vi "输入数据解析.vi"(0 "单个参数补充":dbl, 1 "从板号":dbl=1.0, 2 "主板二维码":string="BNET01", 3 "从板二维码":string="BNET01", 5 "主板引用":refnum<vi>, 7 "从板引用":refnum<vi>, 9 "主板选项":string="三级故障阀值", 11 "枚举":enum16{"主板", "从板"}(ring), 12 "快换":bool caption="快换写入") -> (4 "输出数组":dbl[][](array[numeric]), 6 "数组长度":dbl[](array[numeric]), 8 "循环次数":i32, 10 "命令":u32, 14 "名称":string[](array[string]), 15 "命令序号":u32[](array[numeric]))   [LabVIEW 2013] (continued)
                n6181 = Unbundle By Name(w15990) -> ("项目信息 2"=w15991:refnum<vi>)
                n6182 = property class="Tbl (严格)"(reference=w15991) -> ("Value"=w15989:string[][])  [unwired: 1 in, 2 out]
                n6183 = Multiply(x=w15994, y=2.0) -> (x*y=w15992:dbl)
                n6184 = Index Array(array=w15989, index (col)=1 ("禁用的索引 (列)")) -> (element=w16005:string[])  [unwired: 1 in]
                n6185 = Multiply(x=w15994, y=11.0) -> (x*y=w15995:dbl)
                n6186 = Divide(x=w15992, y=2.0) -> (x/y=w15997:dbl)
                n6187 = Multiply(x=w15992, y=1.5) -> (x*y=w16008:dbl)
                n6188 = Array Subset(array=w16005, index=w15995, length=w15992) -> (w16003:string[])
                n6189 = Round Toward +Infinity(x=w15997) -> (ceil(x): smallest int >= x=w15996:dbl)
                n6190 = Round Toward +Infinity(x=w16008) -> (ceil(x): smallest int >= x=w16000:dbl)
                n6191 = Fract/Exp String To Number(string=w16003) -> (number=w16006:dbl[])  [unwired: 4 out]
                n6192 = for {
                  N: w15996 -> [_]
                  tunnel: w16006 -> [w16032]
                  tunnel: [w16010] -> w16009 mode=indexing
                  i -> [w16031]
                  w16022 = 256.0 ("y")
                  n6193 = Multiply(x=w16031, y=2) -> (x*y=w16029:i32)
                  n6194 = Increment(x=w16029) -> (x+1=w16028:i32)
                  n6195 = Index Array(array=w16032, index #1=w16029, index #2=w16028) -> (element #1=w16023:dbl)  [unwired: 1 out]
                  n6196 = Quotient & Remainder(x=w16023, y=w16022) -> (x-y*floor(x/y)=w16011:dbl, floor(x/y)=w16019:dbl)
                  n6197 = Quotient & Remainder(x=w16023, y=w16022) -> (x-y*floor(x/y)=w16020:dbl, floor(x/y)=w16021:dbl)
                  n6198 = call "二进制解析-8.6.vi"("索引"=4, "数值"=w16019) -> ("低位子数组"=w16015:i32[])  [unwired: 3 out]
                  n6199 = call "二进制解析-8.6.vi"("索引"=4, "数值"=w16021) -> ("低位子数组"=w16018:i32[])  [unwired: 3 out]
                  n6200 = call "二进制解析-8.6.vi"("索引"=4, "数值"=w16020) -> ("低位子数组"=w16016:i32[], "高位子数组"=w16017:i32[])  [unwired: 2 out]
                  n6201 = Insert Into Array(array=w16018, new element=w16017) -> (w16025:i32[])  [unwired: 1 in]
                  n6202 = Insert Into Array(array=w16016, new element=w16015) -> (w16014:i32[])  [unwired: 1 in]
                  n6203 = call "数值二进制转十进制-8.6.vi"("子数组"=w16014) -> ("十进制数值"=w16012:i32)  [unwired: 4 out]
                  n6204 = call "数值二进制转十进制-8.6.vi"("子数组"=w16025) -> ("十进制数值"=w16013:i32)  [unwired: 4 out]
                  n6205 = Build Array(w16013, w16012, w16011) -> (w16010:dbl[])
                }
                n6206 = Reshape Array(w16009, w16000) -> (w15999:dbl[])
              }
              frame 4 {
                n6207 = Unbundle By Name(w16034) -> ("项目信息 2"=w16035:refnum<vi>)
                n6208 = property class="Tbl (严格)"(reference=w16035) -> ("Value"=w16033:string[][])  [unwired: 1 in, 2 out]
                n6209 = Index Array(array=w16033, index (col)=1 ("禁用的索引 (列)")) -> (element=w16040:string[])  [unwired: 1 in]
                n6210 = Multiply(x=w16039, y=6.0) -> (x*y=w16037:dbl)
                n6211 = Array Subset(array=w16040, index=0 ("索引"), length=w16037) -> (w16041:string[])
                n6212 = Fract/Exp String To Number(string=w16041) -> (number=w16038:dbl[])  [unwired: 4 out]
              }
            }
          }
        }
        frame "风机开启温差" {
          n6213 = for {
            N: 1 -> [_]
            tunnel: w16051 -> [w16055]
            tunnel: [w16058] -> w16050 mode=indexing
            tunnel: [w16057] -> w16049 mode=indexing
            tunnel: [w16056] -> w16048 mode=indexing
            tunnel: w16047 -> [w16054]
            i -> [w16059]
            n6214 = case shown="0, 默认" w16059 {
              tunnel: w16054 -> [w16074 w16080 w16121 w16165 w16209]
              tunnel: w16055 -> [_ w16084 w16125 w16169 w16214]
              tunnel: [w16062 w16085 w16130 w16174 w16213] -> w16058
              tunnel: [7.0 w16086 w16131 w16175 w16212] -> w16057
              tunnel: [u32 5 ("命令序号") u32 2 ("命令序号") u32 3 ("命令序号") u32 4 ("命令序号") u32 1 ("命令序号")] -> w16056
              frame 0, Default {
                w16060 = 255 ("高字节1")
                n6215 = Unbundle By Name(w16074) -> ("加热控制参数"=w16075:refnum<vi>)
                n6216 = property class="Clust (严格)"(reference=w16075) -> ("Value"=w16073:T5)  [unwired: 1 in, 2 out]
                n6217 = Unbundle(w16073) -> ("风机开启温度"=w16068:dbl, "风机关闭温度"=w16067:dbl, "加热开启温度"=w16064:dbl, "加热关闭温度"=w16063:dbl, "风机开启温差"=w16061:dbl)  [unwired: 2 out]
                n6218 = call "输入分辨率计算-EV05.vi"("1字节?"=TRUE, "数值 2"=w16063, "数值"=w16064, "偏移量"=-40.0, "分辨率"=1.0) -> ()  [unwired: 7 out]
                n6219 = call "输入分辨率计算-EV05.vi"("1字节?"=TRUE, "数值 2"=w16067, "数值"=w16068, "偏移量"=-40.0, "分辨率"=1.0) -> ()  [unwired: 7 out]
                n6220 = Build Array(w16060, w16060, w16061, w16060, w16060, w16060, w16060) -> (w16062:dbl[])
              }
              frame 1 {
                # "电压起始值"
                n6221 = Unbundle By Name(w16080) -> ("项目信息 2"=w16079:refnum<vi>)
                n6222 = property class="Tbl (严格)"(reference=w16079) -> ("Value"=w16078:string[][])  [unwired: 1 in, 2 out]
                n6223 = Index Array(array=w16078, index (col)=1 ("禁用的索引 (列)")) -> (element=w16092:string[])  [unwired: 1 in]
                n6224 = Multiply(x=w16084, y=6.0) -> (x*y=w16088:dbl)
                n6225 = Divide(x=w16084, y=2.0) -> (x/y=w16082:dbl)
                n6226 = Multiply(x=w16084, y=1.5) -> (x*y=w16095:dbl)
                n6227 = Array Subset(array=w16092, index=w16088, length=w16084) -> (w16090:string[])
                n6228 = Round Toward +Infinity(x=w16082) -> (ceil(x): smallest int >= x=w16081:dbl)
                n6229 = Round Toward +Infinity(x=w16095) -> (ceil(x): smallest int >= x=w16086:dbl)
                n6230 = Fract/Exp String To Number(string=w16090) -> (number=w16093:dbl[])  [unwired: 4 out]
                n6231 = for {
                  N: w16081 -> [_]
                  tunnel: w16093 -> [w16119]
                  tunnel: [w16097] -> w16096 mode=indexing
                  i -> [w16118]
                  w16109 = 256.0 ("y")
                  n6232 = Multiply(x=w16118, y=2) -> (x*y=w16116:i32)
                  n6233 = Increment(x=w16116) -> (x+1=w16115:i32)
                  n6234 = Index Array(array=w16119, index #1=w16116, index #2=w16115) -> (element #1=w16110:dbl)  [unwired: 1 out]
                  n6235 = Quotient & Remainder(x=w16110, y=w16109) -> (x-y*floor(x/y)=w16098:dbl, floor(x/y)=w16106:dbl)
                  n6236 = Quotient & Remainder(x=w16110, y=w16109) -> (x-y*floor(x/y)=w16107:dbl, floor(x/y)=w16108:dbl)
                  n6237 = call "二进制解析-8.6.vi"("索引"=4, "数值"=w16106) -> ("低位子数组"=w16102:i32[])  [unwired: 3 out]
                  n6238 = call "二进制解析-8.6.vi"("索引"=4, "数值"=w16108) -> ("低位子数组"=w16105:i32[])  [unwired: 3 out]
                  n6239 = call "二进制解析-8.6.vi"("索引"=4, "数值"=w16107) -> ("低位子数组"=w16103:i32[], "高位子数组"=w16104:i32[])  [unwired: 2 out]
                  n6240 = Insert Into Array(array=w16105, new element=w16104) -> (w16112:i32[])  [unwired: 1 in]
                  n6241 = Insert Into Array(array=w16103, new element=w16102) -> (w16101:i32[])  [unwired: 1 in]
                  n6242 = call "数值二进制转十进制-8.6.vi"("子数组"=w16101) -> ("十进制数值"=w16099:i32)  [unwired: 4 out]
                  n6243 = call "数值二进制转十进制-8.6.vi"("子数组"=w16112) -> ("十进制数值"=w16100:i32)  [unwired: 4 out]
                  n6244 = Build Array(w16100, w16099, w16098) -> (w16097:dbl[])
                }
                n6245 = Reshape Array(w16096, w16086) -> (w16085:dbl[])
              }
              frame 2 {
                # "电压起始值"
                n6246 = Unbundle By Name(w16121) -> ("项目信息 2"=w16122:refnum<vi>)
                n6247 = property class="Tbl (严格)"(reference=w16122) -> ("Value"=w16120:string[][])  [unwired: 1 in, 2 out]
                n6248 = Multiply(x=w16125, y=5.0) -> (x*y=w16123:dbl)
                n6249 = Index Array(array=w16120, index (col)=1 ("禁用的索引 (列)")) -> (element=w16136:string[])  [unwired: 1 in]
                n6250 = Multiply(x=w16125, y=7.0) -> (x*y=w16126:dbl)
                n6251 = Divide(x=w16123, y=2.0) -> (x/y=w16128:dbl)
                n6252 = Multiply(x=w16123, y=1.5) -> (x*y=w16139:dbl)
                n6253 = Array Subset(array=w16136, index=w16126, length=w16123) -> (w16134:string[])
                n6254 = Round Toward +Infinity(x=w16128) -> (ceil(x): smallest int >= x=w16127:dbl)
                n6255 = Round Toward +Infinity(x=w16139) -> (ceil(x): smallest int >= x=w16131:dbl)
                n6256 = Fract/Exp String To Number(string=w16134) -> (number=w16137:dbl[])  [unwired: 4 out]
                n6257 = for {
                  N: w16127 -> [_]
                  tunnel: w16137 -> [w16163]
                  tunnel: [w16141] -> w16140 mode=indexing
                  i -> [w16162]
                  w16153 = 256.0 ("y")
                  n6258 = Multiply(x=w16162, y=2) -> (x*y=w16160:i32)
                  n6259 = Increment(x=w16160) -> (x+1=w16159:i32)
                  n6260 = Index Array(array=w16163, index #1=w16160, index #2=w16159) -> (element #1=w16154:dbl)  [unwired: 1 out]
                  n6261 = Quotient & Remainder(x=w16154, y=w16153) -> (x-y*floor(x/y)=w16142:dbl, floor(x/y)=w16150:dbl)
                  n6262 = Quotient & Remainder(x=w16154, y=w16153) -> (x-y*floor(x/y)=w16151:dbl, floor(x/y)=w16152:dbl)
                  n6263 = call "二进制解析-8.6.vi"("索引"=4, "数值"=w16150) -> ("低位子数组"=w16146:i32[])  [unwired: 3 out]
                  n6264 = call "二进制解析-8.6.vi"("索引"=4, "数值"=w16152) -> ("低位子数组"=w16149:i32[])  [unwired: 3 out]
                  n6265 = call "二进制解析-8.6.vi"("索引"=4, "数值"=w16151) -> ("低位子数组"=w16147:i32[], "高位子数组"=w16148:i32[])  [unwired: 2 out]
                  n6266 = Insert Into Array(array=w16149, new element=w16148) -> (w16156:i32[])  [unwired: 1 in]
                  n6267 = Insert Into Array(array=w16147, new element=w16146) -> (w16145:i32[])  [unwired: 1 in]
                  n6268 = call "数值二进制转十进制-8.6.vi"("子数组"=w16145) -> ("十进制数值"=w16143:i32)  [unwired: 4 out]
                  n6269 = call "数值二进制转十进制-8.6.vi"("子数组"=w16156) -> ("十进制数值"=w16144:i32)  [unwired: 4 out]
                  n6270 = Build Array(w16144, w16143, w16142) -> (w16141:dbl[])
                }
                n6271 = Reshape Array(w16140, w16131) -> (w16130:dbl[])
              }
              frame 3 {
                # "电压起始值"
                n6272 = Unbundle By Name(w16165) -> ("项目信息 2"=w16166:refnum<vi>)
                n6273 = property class="Tbl (严格)"(reference=w16166) -> ("Value"=w16164:string[][])  [unwired: 1 in, 2 out]
                n6274 = Multiply(x=w16169, y=2.0) -> (x*y=w16167:dbl)
                n6275 = Index Array(array=w16164, index (col)=1 ("禁用的索引 (列)")) -> (element=w16180:string[])  [unwired: 1 in]
                n6276 = Multiply(x=w16169, y=11.0) -> (x*y=w16170:dbl)
                n6277 = Divide(x=w16167, y=2.0) -> (x/y=w16172:dbl)
                n6278 = Multiply(x=w16167, y=1.5) -> (x*y=w16183:dbl)
                n6279 = Array Subset(array=w16180, index=w16170, length=w16167) -> (w16178:string[])
                n6280 = Round Toward +Infinity(x=w16172) -> (ceil(x): smallest int >= x=w16171:dbl)
                n6281 = Round Toward +Infinity(x=w16183) -> (ceil(x): smallest int >= x=w16175:dbl)
                n6282 = Fract/Exp String To Number(string=w16178) -> (number=w16181:dbl[])  [unwired: 4 out]
                n6283 = for {
                  N: w16171 -> [_]
                  tunnel: w16181 -> [w16207]
                  tunnel: [w16185] -> w16184 mode=indexing
                  i -> [w16206]
                  w16197 = 256.0 ("y")
                  n6284 = Multiply(x=w16206, y=2) -> (x*y=w16204:i32)
                  n6285 = Increment(x=w16204) -> (x+1=w16203:i32)
                  n6286 = Index Array(array=w16207, index #1=w16204, index #2=w16203) -> (element #1=w16198:dbl)  [unwired: 1 out]
                  n6287 = Quotient & Remainder(x=w16198, y=w16197) -> (x-y*floor(x/y)=w16186:dbl, floor(x/y)=w16194:dbl)
                  n6288 = Quotient & Remainder(x=w16198, y=w16197) -> (x-y*floor(x/y)=w16195:dbl, floor(x/y)=w16196:dbl)
                  n6289 = call "二进制解析-8.6.vi"("索引"=4, "数值"=w16194) -> ("低位子数组"=w16190:i32[])  [unwired: 3 out]
                  n6290 = call "二进制解析-8.6.vi"("索引"=4, "数值"=w16196) -> ("低位子数组"=w16193:i32[])  [unwired: 3 out]
                  n6291 = call "二进制解析-8.6.vi"("索引"=4, "数值"=w16195) -> ("低位子数组"=w16191:i32[], "高位子数组"=w16192:i32[])  [unwired: 2 out]
                  n6292 = Insert Into Array(array=w16193, new element=w16192) -> (w16200:i32[])  [unwired: 1 in]
                  n6293 = Insert Into Array(array=w16191, new element=w16190) -> (w16189:i32[])  [unwired: 1 in]
                  n6294 = call "数值二进制转十进制-8.6.vi"("子数组"=w16189) -> ("十进制数值"=w16187:i32)  [unwired: 4 out]
                  n6295 = call "数值二进制转十进制-8.6.vi"("子数组"=w16200) -> ("十进制数值"=w16188:i32)  [unwired: 4 out]
                  n6296 = Build Array(w16188, w16187, w16186) -> (w16185:dbl[])
                }
                n6297 = Reshape Array(w16184, w16175) -> (w16174:dbl[])
              }
              frame 4 {
                n6298 = Unbundle By Name(w16209) -> ("项目信息 2"=w16210:refnum<vi>)
                n6299 = property class="Tbl (严格)"(reference=w16210) -> ("Value"=w16208:string[][])  [unwired: 1 in, 2 out]
                n6300 = Index Array(array=w16208, index (col)=1 ("禁用的索引 (列)")) -> (element=w16215:string[])  [unwired: 1 in]
                n6301 = Multiply(x=w16214, y=6.0) -> (x*y=w16212:dbl)
                n6302 = Array Subset(array=w16215, index=0 ("索引"), length=w16212) -> (w16216:string[])
                n6303 = Fract/Exp String To Number(string=w16216) -> (number=w16213:dbl[])  [unwired: 4 out]
              }
            }
          }
        }
        frame "风机关闭温差" {
          n6304 = for {
            N: 1 -> [_]
            tunnel: w16226 -> [w16230]
            tunnel: [w16233] -> w16225 mode=indexing
            tunnel: [w16232] -> w16224 mode=indexing
            tunnel: [w16231] -> w16223 mode=indexing
            tunnel: w16222 -> [w16229]
            i -> [w16234]
            n6305 = case shown="0, 默认" w16234 {
              tunnel: w16229 -> [w16249 w16255 w16296 w16340 w16384]
              tunnel: w16230 -> [_ w16259 w16300 w16344 w16389]
              tunnel: [w16237 w16260 w16305 w16349 w16388] -> w16233
              tunnel: [7.0 w16261 w16306 w16350 w16387] -> w16232
              tunnel: [u32 5 ("命令序号") u32 2 ("命令序号") u32 3 ("命令序号") u32 4 ("命令序号") u32 1 ("命令序号")] -> w16231
              frame 0, Default {
                w16235 = 255 ("高字节1")
                n6306 = Unbundle By Name(w16249) -> ("加热控制参数"=w16250:refnum<vi>)
                n6307 = property class="Clust (严格)"(reference=w16250) -> ("Value"=w16248:T5)  [unwired: 1 in, 2 out]
                n6308 = Unbundle(w16248) -> ("风机开启温度"=w16243:dbl, "风机关闭温度"=w16242:dbl, "加热开启温度"=w16239:dbl, "加热关闭温度"=w16238:dbl, "风机关闭温差"=w16236:dbl)  [unwired: 2 out]
                n6309 = call "输入分辨率计算-EV05.vi"("1字节?"=TRUE, "数值 2"=w16238, "数值"=w16239, "偏移量"=-40.0, "分辨率"=1.0) -> ()  [unwired: 7 out]
                n6310 = call "输入分辨率计算-EV05.vi"("1字节?"=TRUE, "数值 2"=w16242, "数值"=w16243, "偏移量"=-40.0, "分辨率"=1.0) -> ()  [unwired: 7 out]
                n6311 = Build Array(w16235, w16235, w16235, w16236, w16235, w16235, w16235) -> (w16237:dbl[])
              }
              frame 1 {
                # "电压起始值"
                n6312 = Unbundle By Name(w16255) -> ("项目信息 2"=w16254:refnum<vi>)
                n6313 = property class="Tbl (严格)"(reference=w16254) -> ("Value"=w16253:string[][])  [unwired: 1 in, 2 out]
                n6314 = Index Array(array=w16253, index (col)=1 ("禁用的索引 (列)")) -> (element=w16267:string[])  [unwired: 1 in]
                n6315 = Multiply(x=w16259, y=6.0) -> (x*y=w16263:dbl)
                n6316 = Divide(x=w16259, y=2.0) -> (x/y=w16257:dbl)
                n6317 = Multiply(x=w16259, y=1.5) -> (x*y=w16270:dbl)
                n6318 = Array Subset(array=w16267, index=w16263, length=w16259) -> (w16265:string[])
                n6319 = Round Toward +Infinity(x=w16257) -> (ceil(x): smallest int >= x=w16256:dbl)
                n6320 = Round Toward +Infinity(x=w16270) -> (ceil(x): smallest int >= x=w16261:dbl)
                n6321 = Fract/Exp String To Number(string=w16265) -> (number=w16268:dbl[])  [unwired: 4 out]
                n6322 = for {
                  N: w16256 -> [_]
                  tunnel: w16268 -> [w16294]
                  tunnel: [w16272] -> w16271 mode=indexing
                  i -> [w16293]
                  w16284 = 256.0 ("y")
                  n6323 = Multiply(x=w16293, y=2) -> (x*y=w16291:i32)
                  n6324 = Increment(x=w16291) -> (x+1=w16290:i32)
                  n6325 = Index Array(array=w16294, index #1=w16291, index #2=w16290) -> (element #1=w16285:dbl)  [unwired: 1 out]
                  n6326 = Quotient & Remainder(x=w16285, y=w16284) -> (x-y*floor(x/y)=w16273:dbl, floor(x/y)=w16281:dbl)
                  n6327 = Quotient & Remainder(x=w16285, y=w16284) -> (x-y*floor(x/y)=w16282:dbl, floor(x/y)=w16283:dbl)
                  n6328 = call "二进制解析-8.6.vi"("索引"=4, "数值"=w16281) -> ("低位子数组"=w16277:i32[])  [unwired: 3 out]
                  n6329 = call "二进制解析-8.6.vi"("索引"=4, "数值"=w16283) -> ("低位子数组"=w16280:i32[])  [unwired: 3 out]
                  n6330 = call "二进制解析-8.6.vi"("索引"=4, "数值"=w16282) -> ("低位子数组"=w16278:i32[], "高位子数组"=w16279:i32[])  [unwired: 2 out]
                  n6331 = Insert Into Array(array=w16280, new element=w16279) -> (w16287:i32[])  [unwired: 1 in]
                  n6332 = Insert Into Array(array=w16278, new element=w16277) -> (w16276:i32[])  [unwired: 1 in]
                  n6333 = call "数值二进制转十进制-8.6.vi"("子数组"=w16276) -> ("十进制数值"=w16274:i32)  [unwired: 4 out]
                  n6334 = call "数值二进制转十进制-8.6.vi"("子数组"=w16287) -> ("十进制数值"=w16275:i32)  [unwired: 4 out]
                  n6335 = Build Array(w16275, w16274, w16273) -> (w16272:dbl[])
                }
                n6336 = Reshape Array(w16271, w16261) -> (w16260:dbl[])
              }
              frame 2 {
                # "电压起始值"
                n6337 = Unbundle By Name(w16296) -> ("项目信息 2"=w16297:refnum<vi>)
                n6338 = property class="Tbl (严格)"(reference=w16297) -> ("Value"=w16295:string[][])  [unwired: 1 in, 2 out]
                n6339 = Multiply(x=w16300, y=5.0) -> (x*y=w16298:dbl)
                n6340 = Index Array(array=w16295, index (col)=1 ("禁用的索引 (列)")) -> (element=w16311:string[])  [unwired: 1 in]
                n6341 = Multiply(x=w16300, y=7.0) -> (x*y=w16301:dbl)
                n6342 = Divide(x=w16298, y=2.0) -> (x/y=w16303:dbl)
                n6343 = Multiply(x=w16298, y=1.5) -> (x*y=w16314:dbl)
                n6344 = Array Subset(array=w16311, index=w16301, length=w16298) -> (w16309:string[])
                n6345 = Round Toward +Infinity(x=w16303) -> (ceil(x): smallest int >= x=w16302:dbl)
                n6346 = Round Toward +Infinity(x=w16314) -> (ceil(x): smallest int >= x=w16306:dbl)
                n6347 = Fract/Exp String To Number(string=w16309) -> (number=w16312:dbl[])  [unwired: 4 out]
                n6348 = for {
                  N: w16302 -> [_]
                  tunnel: w16312 -> [w16338]
                  tunnel: [w16316] -> w16315 mode=indexing
                  i -> [w16337]
                  w16328 = 256.0 ("y")
                  n6349 = Multiply(x=w16337, y=2) -> (x*y=w16335:i32)
                  n6350 = Increment(x=w16335) -> (x+1=w16334:i32)
                  n6351 = Index Array(array=w16338, index #1=w16335, index #2=w16334) -> (element #1=w16329:dbl)  [unwired: 1 out]
                  n6352 = Quotient & Remainder(x=w16329, y=w16328) -> (x-y*floor(x/y)=w16317:dbl, floor(x/y)=w16325:dbl)
                  n6353 = Quotient & Remainder(x=w16329, y=w16328) -> (x-y*floor(x/y)=w16326:dbl, floor(x/y)=w16327:dbl)
                  n6354 = call "二进制解析-8.6.vi"("索引"=4, "数值"=w16325) -> ("低位子数组"=w16321:i32[])  [unwired: 3 out]
                  n6355 = call "二进制解析-8.6.vi"("索引"=4, "数值"=w16327) -> ("低位子数组"=w16324:i32[])  [unwired: 3 out]
                  n6356 = call "二进制解析-8.6.vi"("索引"=4, "数值"=w16326) -> ("低位子数组"=w16322:i32[], "高位子数组"=w16323:i32[])  [unwired: 2 out]
                  n6357 = Insert Into Array(array=w16324, new element=w16323) -> (w16331:i32[])  [unwired: 1 in]
                  n6358 = Insert Into Array(array=w16322, new element=w16321) -> (w16320:i32[])  [unwired: 1 in]
                  n6359 = call "数值二进制转十进制-8.6.vi"("子数组"=w16320) -> ("十进制数值"=w16318:i32)  [unwired: 4 out]
                  n6360 = call "数值二进制转十进制-8.6.vi"("子数组"=w16331) -> ("十进制数值"=w16319:i32)  [unwired: 4 out]
                  n6361 = Build Array(w16319, w16318, w16317) -> (w16316:dbl[])
                }
                n6362 = Reshape Array(w16315, w16306) -> (w16305:dbl[])
              }
              frame 3 {
                # "电压起始值"
                n6363 = Unbundle By Name(w16340) -> ("项目信息 2"=w16341:refnum<vi>)
                n6364 = property class="Tbl (严格)"(reference=w16341) -> ("Value"=w16339:string[][])  [unwired: 1 in, 2 out]
                n6365 = Multiply(x=w16344, y=2.0) -> (x*y=w16342:dbl)
                n6366 = Index Array(array=w16339, index (col)=1 ("禁用的索引 (列)")) -> (element=w16355:string[])  [unwired: 1 in]
                n6367 = Multiply(x=w16344, y=11.0) -> (x*y=w16345:dbl)
                n6368 = Divide(x=w16342, y=2.0) -> (x/y=w16347:dbl)
                n6369 = Multiply(x=w16342, y=1.5) -> (x*y=w16358:dbl)
                n6370 = Array Subset(array=w16355, index=w16345, length=w16342) -> (w16353:string[])
                n6371 = Round Toward +Infinity(x=w16347) -> (ceil(x): smallest int >= x=w16346:dbl)
                n6372 = Round Toward +Infinity(x=w16358) -> (ceil(x): smallest int >= x=w16350:dbl)
                n6373 = Fract/Exp String To Number(string=w16353) -> (number=w16356:dbl[])  [unwired: 4 out]
                n6374 = for {
                  N: w16346 -> [_]
                  tunnel: w16356 -> [w16382]
                  tunnel: [w16360] -> w16359 mode=indexing
                  i -> [w16381]
                  w16372 = 256.0 ("y")
                  n6375 = Multiply(x=w16381, y=2) -> (x*y=w16379:i32)
                  n6376 = Increment(x=w16379) -> (x+1=w16378:i32)
                  n6377 = Index Array(array=w16382, index #1=w16379, index #2=w16378) -> (element #1=w16373:dbl)  [unwired: 1 out]
                  n6378 = Quotient & Remainder(x=w16373, y=w16372) -> (x-y*floor(x/y)=w16361:dbl, floor(x/y)=w16369:dbl)
                  n6379 = Quotient & Remainder(x=w16373, y=w16372) -> (x-y*floor(x/y)=w16370:dbl, floor(x/y)=w16371:dbl)
                  n6380 = call "二进制解析-8.6.vi"("索引"=4, "数值"=w16369) -> ("低位子数组"=w16365:i32[])  [unwired: 3 out]
                  n6381 = call "二进制解析-8.6.vi"("索引"=4, "数值"=w16371) -> ("低位子数组"=w16368:i32[])  [unwired: 3 out]
                  n6382 = call "二进制解析-8.6.vi"("索引"=4, "数值"=w16370) -> ("低位子数组"=w16366:i32[], "高位子数组"=w16367:i32[])  [unwired: 2 out]
                  n6383 = Insert Into Array(array=w16368, new element=w16367) -> (w16375:i32[])  [unwired: 1 in]
                  n6384 = Insert Into Array(array=w16366, new element=w16365) -> (w16364:i32[])  [unwired: 1 in]
                  n6385 = call "数值二进制转十进制-8.6.vi"("子数组"=w16364) -> ("十进制数值"=w16362:i32)  [unwired: 4 out]
                  n6386 = call "数值二进制转十进制-8.6.vi"("子数组"=w16375) -> ("十进制数值"=w16363:i32)  [unwired: 4 out]
                  n6387 = Build Array(w16363, w16362, w16361) -> (w16360:dbl[])
                }
                n6388 = Reshape Array(w16359, w16350) -> (w16349:dbl[])
              }
              frame 4 {
                n6389 = Unbundle By Name(w16384) -> ("项目信息 2"=w16385:refnum<vi>)
                n6390 = property class="Tbl (严格)"(reference=w16385) -> ("Value"=w16383:string[][])  [unwired: 1 in, 2 out]
                n6391 = Index Array(array=w16383, index (col)=1 ("禁用的索引 (列)")) -> (element=w16390:string[])  [unwired: 1 in]
                n6392 = Multiply(x=w16389, y=6.0) -> (x*y=w16387:dbl)
                n6393 = Array Subset(array=w16390, index=0 ("索引"), length=w16387) -> (w16391:string[])
                n6394 = Fract/Exp String To Number(string=w16391) -> (number=w16388:dbl[])  [unwired: 4 out]
              }
            }
          }
        }
        frame "加热关闭温差" {
          n6395 = for {
            N: 1 -> [_]
            tunnel: w16401 -> [w16405]
            tunnel: [w16408] -> w16400 mode=indexing
            tunnel: [w16407] -> w16399 mode=indexing
            tunnel: [w16406] -> w16398 mode=indexing
            tunnel: w16397 -> [w16404]
            i -> [w16409]
            n6396 = case shown="0, 默认" w16409 {
              tunnel: w16404 -> [w16424 w16430 w16471 w16515 w16559]
              tunnel: w16405 -> [_ w16434 w16475 w16519 w16564]
              tunnel: [w16412 w16435 w16480 w16524 w16563] -> w16408
              tunnel: [7.0 w16436 w16481 w16525 w16562] -> w16407
              tunnel: [u32 5 ("命令序号") u32 2 ("命令序号") u32 3 ("命令序号") u32 4 ("命令序号") u32 1 ("命令序号")] -> w16406
              frame 0, Default {
                w16411 = 255 ("高字节1")
                n6397 = Unbundle By Name(w16424) -> ("加热控制参数"=w16425:refnum<vi>)
                n6398 = property class="Clust (严格)"(reference=w16425) -> ("Value"=w16423:T5)  [unwired: 1 in, 2 out]
                n6399 = Unbundle(w16423) -> ("风机开启温度"=w16418:dbl, "风机关闭温度"=w16417:dbl, "加热开启温度"=w16414:dbl, "加热关闭温度"=w16413:dbl, "加热关闭温差"=w16410:dbl)  [unwired: 2 out]
                n6400 = call "输入分辨率计算-EV05.vi"("1字节?"=TRUE, "数值 2"=w16413, "数值"=w16414, "偏移量"=-40.0, "分辨率"=1.0) -> ()  [unwired: 7 out]
                n6401 = call "输入分辨率计算-EV05.vi"("1字节?"=TRUE, "数值 2"=w16417, "数值"=w16418, "偏移量"=-40.0, "分辨率"=1.0) -> ()  [unwired: 7 out]
                n6402 = Build Array(w16411, w16411, w16411, w16411, w16411, w16411, w16410) -> (w16412:dbl[])
              }
              frame 1 {
                # "电压起始值"
                n6403 = Unbundle By Name(w16430) -> ("项目信息 2"=w16429:refnum<vi>)
                n6404 = property class="Tbl (严格)"(reference=w16429) -> ("Value"=w16428:string[][])  [unwired: 1 in, 2 out]
                n6405 = Index Array(array=w16428, index (col)=1 ("禁用的索引 (列)")) -> (element=w16442:string[])  [unwired: 1 in]
                n6406 = Multiply(x=w16434, y=6.0) -> (x*y=w16438:dbl)
                n6407 = Divide(x=w16434, y=2.0) -> (x/y=w16432:dbl)
                n6408 = Multiply(x=w16434, y=1.5) -> (x*y=w16445:dbl)
                n6409 = Array Subset(array=w16442, index=w16438, length=w16434) -> (w16440:string[])
                n6410 = Round Toward +Infinity(x=w16432) -> (ceil(x): smallest int >= x=w16431:dbl)
                n6411 = Round Toward +Infinity(x=w16445) -> (ceil(x): smallest int >= x=w16436:dbl)
                n6412 = Fract/Exp String To Number(string=w16440) -> (number=w16443:dbl[])  [unwired: 4 out]
                n6413 = for {
                  N: w16431 -> [_]
                  tunnel: w16443 -> [w16469]
                  tunnel: [w16447] -> w16446 mode=indexing
                  i -> [w16468]
                  w16459 = 256.0 ("y")
                  n6414 = Multiply(x=w16468, y=2) -> (x*y=w16466:i32)
                  n6415 = Increment(x=w16466) -> (x+1=w16465:i32)
                  n6416 = Index Array(array=w16469, index #1=w16466, index #2=w16465) -> (element #1=w16460:dbl)  [unwired: 1 out]
                  n6417 = Quotient & Remainder(x=w16460, y=w16459) -> (x-y*floor(x/y)=w16448:dbl, floor(x/y)=w16456:dbl)
                  n6418 = Quotient & Remainder(x=w16460, y=w16459) -> (x-y*floor(x/y)=w16457:dbl, floor(x/y)=w16458:dbl)
                  n6419 = call "二进制解析-8.6.vi"("索引"=4, "数值"=w16456) -> ("低位子数组"=w16452:i32[])  [unwired: 3 out]
                  n6420 = call "二进制解析-8.6.vi"("索引"=4, "数值"=w16458) -> ("低位子数组"=w16455:i32[])  [unwired: 3 out]
                  n6421 = call "二进制解析-8.6.vi"("索引"=4, "数值"=w16457) -> ("低位子数组"=w16453:i32[], "高位子数组"=w16454:i32[])  [unwired: 2 out]
                  n6422 = Insert Into Array(array=w16455, new element=w16454) -> (w16462:i32[])  [unwired: 1 in]
                  n6423 = Insert Into Array(array=w16453, new element=w16452) -> (w16451:i32[])  [unwired: 1 in]
                  n6424 = call "数值二进制转十进制-8.6.vi"("子数组"=w16451) -> ("十进制数值"=w16449:i32)  [unwired: 4 out]
                  n6425 = call "数值二进制转十进制-8.6.vi"("子数组"=w16462) -> ("十进制数值"=w16450:i32)  [unwired: 4 out]
                  n6426 = Build Array(w16450, w16449, w16448) -> (w16447:dbl[])
                }
                n6427 = Reshape Array(w16446, w16436) -> (w16435:dbl[])
              }
              frame 2 {
                # "电压起始值"
                n6428 = Unbundle By Name(w16471) -> ("项目信息 2"=w16472:refnum<vi>)
                n6429 = property class="Tbl (严格)"(reference=w16472) -> ("Value"=w16470:string[][])  [unwired: 1 in, 2 out]
                n6430 = Multiply(x=w16475, y=5.0) -> (x*y=w16473:dbl)
                n6431 = Index Array(array=w16470, index (col)=1 ("禁用的索引 (列)")) -> (element=w16486:string[])  [unwired: 1 in]
                n6432 = Multiply(x=w16475, y=7.0) -> (x*y=w16476:dbl)
                n6433 = Divide(x=w16473, y=2.0) -> (x/y=w16478:dbl)
                n6434 = Multiply(x=w16473, y=1.5) -> (x*y=w16489:dbl)
                n6435 = Array Subset(array=w16486, index=w16476, length=w16473) -> (w16484:string[])
                n6436 = Round Toward +Infinity(x=w16478) -> (ceil(x): smallest int >= x=w16477:dbl)
                n6437 = Round Toward +Infinity(x=w16489) -> (ceil(x): smallest int >= x=w16481:dbl)
                n6438 = Fract/Exp String To Number(string=w16484) -> (number=w16487:dbl[])  [unwired: 4 out]
                n6439 = for {
                  N: w16477 -> [_]
                  tunnel: w16487 -> [w16513]
                  tunnel: [w16491] -> w16490 mode=indexing
                  i -> [w16512]
                  w16503 = 256.0 ("y")
                  n6440 = Multiply(x=w16512, y=2) -> (x*y=w16510:i32)
                  n6441 = Increment(x=w16510) -> (x+1=w16509:i32)
                  n6442 = Index Array(array=w16513, index #1=w16510, index #2=w16509) -> (element #1=w16504:dbl)  [unwired: 1 out]
                  n6443 = Quotient & Remainder(x=w16504, y=w16503) -> (x-y*floor(x/y)=w16492:dbl, floor(x/y)=w16500:dbl)
                  n6444 = Quotient & Remainder(x=w16504, y=w16503) -> (x-y*floor(x/y)=w16501:dbl, floor(x/y)=w16502:dbl)
                  n6445 = call "二进制解析-8.6.vi"("索引"=4, "数值"=w16500) -> ("低位子数组"=w16496:i32[])  [unwired: 3 out]
                  n6446 = call "二进制解析-8.6.vi"("索引"=4, "数值"=w16502) -> ("低位子数组"=w16499:i32[])  [unwired: 3 out]
                  n6447 = call "二进制解析-8.6.vi"("索引"=4, "数值"=w16501) -> ("低位子数组"=w16497:i32[], "高位子数组"=w16498:i32[])  [unwired: 2 out]
                  n6448 = Insert Into Array(array=w16499, new element=w16498) -> (w16506:i32[])  [unwired: 1 in]
                  n6449 = Insert Into Array(array=w16497, new element=w16496) -> (w16495:i32[])  [unwired: 1 in]
                  n6450 = call "数值二进制转十进制-8.6.vi"("子数组"=w16495) -> ("十进制数值"=w16493:i32)  [unwired: 4 out]
                  n6451 = call "数值二进制转十进制-8.6.vi"("子数组"=w16506) -> ("十进制数值"=w16494:i32)  [unwired: 4 out]
                  n6452 = Build Array(w16494, w16493, w16492) -> (w16491:dbl[])
                }
                n6453 = Reshape Array(w16490, w16481) -> (w16480:dbl[])
              }
              frame 3 {
                # "电压起始值"
                n6454 = Unbundle By Name(w16515) -> ("项目信息 2"=w16516:refnum<vi>)
                n6455 = property class="Tbl (严格)"(reference=w16516) -> ("Value"=w16514:string[][])  [unwired: 1 in, 2 out]
                n6456 = Multiply(x=w16519, y=2.0) -> (x*y=w16517:dbl)
                n6457 = Index Array(array=w16514, index (col)=1 ("禁用的索引 (列)")) -> (element=w16530:string[])  [unwired: 1 in]
                n6458 = Multiply(x=w16519, y=11.0) -> (x*y=w16520:dbl)
                n6459 = Divide(x=w16517, y=2.0) -> (x/y=w16522:dbl)
                n6460 = Multiply(x=w16517, y=1.5) -> (x*y=w16533:dbl)
                n6461 = Array Subset(array=w16530, index=w16520, length=w16517) -> (w16528:string[])
                n6462 = Round Toward +Infinity(x=w16522) -> (ceil(x): smallest int >= x=w16521:dbl)
                n6463 = Round Toward +Infinity(x=w16533) -> (ceil(x): smallest int >= x=w16525:dbl)
                n6464 = Fract/Exp String To Number(string=w16528) -> (number=w16531:dbl[])  [unwired: 4 out]
                n6465 = for {
                  N: w16521 -> [_]
                  tunnel: w16531 -> [w16557]
                  tunnel: [w16535] -> w16534 mode=indexing
                  i -> [w16556]
                  w16547 = 256.0 ("y")
                  n6466 = Multiply(x=w16556, y=2) -> (x*y=w16554:i32)
                  n6467 = Increment(x=w16554) -> (x+1=w16553:i32)
                  n6468 = Index Array(array=w16557, index #1=w16554, index #2=w16553) -> (element #1=w16548:dbl)  [unwired: 1 out]
                  n6469 = Quotient & Remainder(x=w16548, y=w16547) -> (x-y*floor(x/y)=w16536:dbl, floor(x/y)=w16544:dbl)
                  n6470 = Quotient & Remainder(x=w16548, y=w16547) -> (x-y*floor(x/y)=w16545:dbl, floor(x/y)=w16546:dbl)
                  n6471 = call "二进制解析-8.6.vi"("索引"=4, "数值"=w16544) -> ("低位子数组"=w16540:i32[])  [unwired: 3 out]
                  n6472 = call "二进制解析-8.6.vi"("索引"=4, "数值"=w16546) -> ("低位子数组"=w16543:i32[])  [unwired: 3 out]
                  n6473 = call "二进制解析-8.6.vi"("索引"=4, "数值"=w16545) -> ("低位子数组"=w16541:i32[], "高位子数组"=w16542:i32[])  [unwired: 2 out]
                  n6474 = Insert Into Array(array=w16543, new element=w16542) -> (w16550:i32[])  [unwired: 1 in]
                  n6475 = Insert Into Array(array=w16541, new element=w16540) -> (w16539:i32[])  [unwired: 1 in]
                  n6476 = call "数值二进制转十进制-8.6.vi"("子数组"=w16539) -> ("十进制数值"=w16537:i32)  [unwired: 4 out]
                  n6477 = call "数值二进制转十进制-8.6.vi"("子数组"=w16550) -> ("十进制数值"=w16538:i32)  [unwired: 4 out]
                  n6478 = Build Array(w16538, w16537, w16536) -> (w16535:dbl[])
                }
                n6479 = Reshape Array(w16534, w16525) -> (w16524:dbl[])
              }
              frame 4 {
                n6480 = Unbundle By Name(w16559) -> ("项目信息 2"=w16560:refnum<vi>)
                n6481 = property class="Tbl (严格)"(reference=w16560) -> ("Value"=w16558:string[][])  [unwired: 1 in, 2 out]
                n6482 = Index Array(array=w16558, index (col)=1 ("禁用的索引 (列)")) -> (element=w16565:string[])  [unwired: 1 in]
                n6483 = Multiply(x=w16564, y=6.0) -> (x*y=w16562:dbl)
                n6484 = Array Subset(array=w16565, index=0 ("索引"), length=w16562) -> (w16566:string[])
                n6485 = Fract/Exp String To Number(string=w16566) -> (number=w16563:dbl[])  [unwired: 4 out]
              }
            }
          }
        }
        frame "一级故障阀值" {
          n6486 = Unbundle By Name(w16575) -> ("一级故障(从板)"=w16576:refnum<vi>)
          n6487 = property class="Clust (严格)"(reference=w16576) -> ("Value"=w16574:T8)  [unwired: 1 in, 2 out]
          n6488 = for {
            N: 7 -> [_]
            tunnel: w16574 -> [w16587]
            shift-right: [w16586] -> w16578
            shift-left: dbl[] [] -> [w16585]
            tunnel: 0.001 ("分辨率") -> [w16583]
            i -> [w16588]
            n6489 = case shown="0, 默认" w16588 {
              tunnel: w16587 -> [w16591 w16598 w16604 w16611 w16618 w16625 w16633]
              tunnel: [w16592 w16599 w16605 w16613 w16620 w16626 w16634] -> w16584
              tunnel: w16583 -> [w16589 w16596 _ _ _ _ _]
              frame 0, Default {
                # "电压过高"
                n6490 = Unbundle By Name(w16591) -> ("电压过高"=w16590:dbl)
                n6491 = call "输入分辨率计算-EV05.vi"("1字节?"=FALSE, "数值"=w16590, "分辨率"=w16589) -> ("低字节"=w16593:dbl, "高字节1"=w16594:dbl)  [unwired: 2 in, 5 out]
                n6492 = Build Array(w16594, w16593) -> (w16592:dbl[])
              }
              frame 1 {
                # "电压过低"
                n6493 = Unbundle By Name(w16598) -> ("电压过低"=w16597:dbl)
                n6494 = call "输入分辨率计算-EV05.vi"("1字节?"=FALSE, "数值"=w16597, "分辨率"=w16596) -> ("低字节"=w16600:dbl, "高字节1"=w16601:dbl)  [unwired: 2 in, 5 out]
                n6495 = Build Array(w16601, w16600) -> (w16599:dbl[])
              }
              frame 2 {
                # "电压不均衡"
                n6496 = Unbundle By Name(w16604) -> ("电压不均衡(V)"=w16603:dbl)
                n6497 = call "输入分辨率计算-EV05.vi"("1字节?"=FALSE, "数值"=w16603, "分辨率"=0.001) -> ("低字节"=w16606:dbl, "高字节1"=w16607:dbl)  [unwired: 2 in, 5 out]
                n6498 = Build Array(w16607, w16606) -> (w16605:dbl[])
              }
              frame 3 {
                # "温度过高"
                n6499 = Unbundle By Name(w16611) -> ("温度过高"=w16610:dbl)
                n6500 = call "输入分辨率计算-EV05.vi"("1字节?"=TRUE, "数值"=w16610, "偏移量"=-40.0, "分辨率"=1.0) -> ("高字节1"=w16614:dbl)  [unwired: 1 in, 6 out]
                n6501 = Build Array(w16614) -> (w16613:dbl[])
              }
              frame 4 {
                # "温度过低"
                n6502 = Unbundle By Name(w16618) -> ("温度过低"=w16617:dbl)
                n6503 = call "输入分辨率计算-EV05.vi"("1字节?"=TRUE, "数值"=w16617, "偏移量"=-40.0, "分辨率"=1.0) -> ("高字节1"=w16621:dbl)  [unwired: 1 in, 6 out]
                n6504 = Build Array(w16621) -> (w16620:dbl[])
              }
              frame 5 {
                # "温度不均衡"
                n6505 = Unbundle By Name(w16625) -> ("温度不均衡"=w16624:dbl)
                n6506 = call "输入分辨率计算-EV05.vi"("1字节?"=TRUE, "数值"=w16624, "分辨率"=1.0) -> ("高字节1"=w16627:dbl)  [unwired: 2 in, 6 out]
                n6507 = Build Array(w16627) -> (w16626:dbl[])
              }
              frame 6 {
                # "SOC过低"
                n6508 = Unbundle By Name(w16633) -> ("SOC过低"=w16632:dbl)
                n6509 = call "输入分辨率计算-EV05.vi"("1字节?"=FALSE, "数值"=w16632, "分辨率"=0.1) -> ("低字节"=w16630:dbl, "高字节1"=w16631:dbl)  [unwired: 2 in, 5 out]
                n6510 = Build Array(w16631, w16630) -> (w16634:dbl[])
              }
            }
            n6511 = Insert Into Array(array=w16585, new element=w16584) -> (w16586:dbl[])  [unwired: 1 in]
          }
          n6512 = Build Array(w16578) -> (w16577:dbl[][])
        }
        frame "电压过高" {
          n6513 = Unbundle By Name(w16641) -> ("一级故障(从板)"=w16642:refnum<vi>)
          n6514 = property class="Clust (严格)"(reference=w16642) -> ("Value"=w16640:T8)  [unwired: 1 in, 2 out]
          n6515 = for {
            N: 7 -> [_]
            tunnel: w16640 -> [w16652]
            shift-right: [w16651] -> w16644
            shift-left: dbl[] [] -> [w16650]
            i -> [w16653]
            n6516 = case shown="0, 默认" w16653 {
              tunnel: w16652 -> [w16654 w16665 w16676 w16687 w16697 w16707 w16718]
              tunnel: [w16655 w16666 w16677 w16688 w16698 w16708 w16719] -> w16649
              frame 0, Default {
                # "电压过高"
                n6517 = disable-structure shown="启用" {
                  disable-tunnel: [w16661 w16664] -> w16657
                  disable-tunnel: [w16660 w16664] -> w16656
                  disable-tunnel: w16654 -> [w16659 _]
                  frame Enabled {
                    n6518 = Unbundle By Name(w16659) -> ("电压过高"=w16658:dbl)
                    n6519 = call "输入分辨率计算-EV05.vi"("1字节?"=FALSE, "数值"=w16658, "分辨率"=0.001) -> ("低字节"=w16660:dbl, "高字节1"=w16661:dbl)  [unwired: 2 in, 5 out]
                  }
                  frame Disabled {
                    w16664 = 255 ("高字节1")
                  }
                }
                n6520 = Build Array(w16657, w16656) -> (w16655:dbl[])
              }
              frame 1 {
                # "电压过低"
                n6521 = disable-structure shown="启用" {
                  disable-tunnel: [w16672 w16675] -> w16668
                  disable-tunnel: [w16671 w16675] -> w16667
                  disable-tunnel: w16665 -> [w16670 _]
                  frame Disabled {
                    n6522 = Unbundle By Name(w16670) -> ("电压过低"=w16669:dbl)
                    n6523 = call "输入分辨率计算-EV05.vi"("1字节?"=FALSE, "数值"=w16669, "分辨率"=0.1) -> ("低字节"=w16671:dbl, "高字节1"=w16672:dbl)  [unwired: 2 in, 5 out]
                  }
                  frame Enabled {
                    w16675 = 255 ("高字节1")
                  }
                }
                n6524 = Build Array(w16668, w16667) -> (w16666:i32[])
              }
              frame 2 {
                # "电压不均衡"
                n6525 = disable-structure shown="启用" {
                  disable-tunnel: [w16683 w16686] -> w16679
                  disable-tunnel: [w16682 w16686] -> w16678
                  disable-tunnel: w16676 -> [w16681 _]
                  frame Disabled {
                    n6526 = Unbundle By Name(w16681) -> ("电压不均衡(V)"=w16680:dbl)
                    n6527 = call "输入分辨率计算-EV05.vi"("1字节?"=FALSE, "数值"=w16680, "分辨率"=0.1) -> ("低字节"=w16682:dbl, "高字节1"=w16683:dbl)  [unwired: 2 in, 5 out]
                  }
                  frame Enabled {
                    w16686 = 255 ("高字节1")
                  }
                }
                n6528 = Build Array(w16679, w16678) -> (w16677:i32[])
              }
              frame 3 {
                # "温度过高"
                n6529 = disable-structure shown="启用" {
                  disable-tunnel: [w16693 255 ("高字节1")] -> w16689
                  disable-tunnel: w16687 -> [w16691 _]
                  frame Disabled {
                    n6530 = Unbundle By Name(w16691) -> ("温度过高"=w16690:dbl)
                    n6531 = call "输入分辨率计算-EV05.vi"("1字节?"=TRUE, "数值"=w16690, "偏移量"=-40.0, "分辨率"=1.0) -> ("高字节1"=w16693:dbl)  [unwired: 1 in, 6 out]
                  }
                  frame Enabled {
                  }
                }
                n6532 = Build Array(w16689) -> (w16688:i32[])
              }
              frame 4 {
                # "温度过低"
                n6533 = disable-structure shown="启用" {
                  disable-tunnel: [w16703 255 ("高字节1")] -> w16699
                  disable-tunnel: w16697 -> [w16701 _]
                  frame Disabled {
                    n6534 = Unbundle By Name(w16701) -> ("温度过低"=w16700:dbl)
                    n6535 = call "输入分辨率计算-EV05.vi"("1字节?"=TRUE, "数值"=w16700, "偏移量"=-40.0, "分辨率"=1.0) -> ("高字节1"=w16703:dbl)  [unwired: 1 in, 6 out]
                  }
                  frame Enabled {
                  }
                }
                n6536 = Build Array(w16699) -> (w16698:i32[])
              }
              frame 5 {
                # "温度不均衡"
                n6537 = disable-structure shown="启用" {
                  disable-tunnel: [w16712 255 ("高字节1")] -> w16709
                  disable-tunnel: w16707 -> [w16711 _]
                  frame Disabled {
                    n6538 = Unbundle By Name(w16711) -> ("温度不均衡"=w16710:dbl)
                    n6539 = call "输入分辨率计算-EV05.vi"("1字节?"=TRUE, "数值"=w16710, "分辨率"=1.0) -> ("高字节1"=w16712:dbl)  [unwired: 2 in, 6 out]
                  }
                  frame Enabled {
                  }
                }
                n6540 = Build Array(w16709) -> (w16708:i32[])
              }
              frame 6 {
                # "SOC过低"
                n6541 = disable-structure shown="启用" {
                  disable-tunnel: w16718 -> [w16735 _]
                  disable-tunnel: [w16721 w16738] -> w16717
                  disable-tunnel: [w16720 w16738] -> w16716
                  frame Disabled {
                    n6542 = Unbundle By Name(w16735) -> ("SOC过低"=w16734:dbl)
                    n6543 = call "输入分辨率计算-EV05.vi"("1字节?"=FALSE, "数值"=w16734, "分辨率"=0.1) -> ("低字节"=w16723:dbl, "高字节1"=w16724:dbl)  [unwired: 2 in, 5 out]
                    n6544 = call "二进制解析-8.6.vi"("索引"=4, "数值"=0) -> ("低位子数组"=w16727:i32[])  [unwired: 3 out]
                    n6545 = call "二进制解析-8.6.vi"("索引"=4, "数值"=w16724) -> ("低位子数组"=w16730:i32[])  [unwired: 3 out]
                    n6546 = call "二进制解析-8.6.vi"("索引"=4, "数值"=w16723) -> ("低位子数组"=w16728:i32[], "高位子数组"=w16729:i32[])  [unwired: 2 out]
                    n6547 = Insert Into Array(array=w16730, new element=w16729) -> (w16732:i32[])  [unwired: 1 in]
                    n6548 = Insert Into Array(array=w16728, new element=w16727) -> (w16726:i32[])  [unwired: 1 in]
                    n6549 = call "数值二进制转十进制-8.6.vi"("子数组"=w16726) -> ("十进制数值"=w16721:i32)  [unwired: 4 out]
                    n6550 = call "数值二进制转十进制-8.6.vi"("子数组"=w16732) -> ("十进制数值"=w16720:i32)  [unwired: 4 out]
                  }
                  frame Enabled {
                    w16738 = 255 ("高字节1")
                  }
                }
                n6551 = Build Array(w16716, w16717) -> (w16719:i32[])
              }
            }
            n6552 = Insert Into Array(array=w16650, new element=w16649) -> (w16651:dbl[])  [unwired: 1 in]
          }
          n6553 = Build Array(w16644) -> (w16643:dbl[][])
        }
        frame "电压过高(2)" {
          n6554 = Unbundle By Name(w16743) -> ("二级故障(从板)"=w16744:refnum<vi>)
          n6555 = property class="Clust (严格)"(reference=w16744) -> ("Value"=w16742:T8)  [unwired: 1 in, 2 out]
          n6556 = for {
            N: 7 -> [_]
            tunnel: w16742 -> [w16754]
            shift-right: [w16753] -> w16746
            shift-left: dbl[] [] -> [w16752]
            i -> [w16755]
            n6557 = case shown="0, 默认" w16755 {
              tunnel: w16754 -> [w16756 w16767 w16778 w16789 w16799 w16809 w16820]
              tunnel: [w16757 w16768 w16779 w16790 w16800 w16810 w16821] -> w16751
              frame 0, Default {
                # "电压过高"
                n6558 = disable-structure shown="启用" {
                  disable-tunnel: [w16763 w16766] -> w16759
                  disable-tunnel: [w16762 w16766] -> w16758
                  disable-tunnel: w16756 -> [w16761 _]
                  frame Enabled {
                    n6559 = Unbundle By Name(w16761) -> ("电压过高"=w16760:dbl)
                    n6560 = call "输入分辨率计算-EV05.vi"("1字节?"=FALSE, "数值"=w16760, "分辨率"=0.001) -> ("低字节"=w16762:dbl, "高字节1"=w16763:dbl)  [unwired: 2 in, 5 out]
                  }
                  frame Disabled {
                    w16766 = 255 ("高字节1")
                  }
                }
                n6561 = Build Array(w16759, w16758) -> (w16757:dbl[])
              }
              frame 1 {
                # "电压过低"
                n6562 = disable-structure shown="启用" {
                  disable-tunnel: [w16774 w16777] -> w16770
                  disable-tunnel: [w16773 w16777] -> w16769
                  disable-tunnel: w16767 -> [w16772 _]
                  frame Disabled {
                    n6563 = Unbundle By Name(w16772) -> ("电压过低"=w16771:dbl)
                    n6564 = call "输入分辨率计算-EV05.vi"("1字节?"=FALSE, "数值"=w16771, "分辨率"=0.1) -> ("低字节"=w16773:dbl, "高字节1"=w16774:dbl)  [unwired: 2 in, 5 out]
                  }
                  frame Enabled {
                    w16777 = 255 ("高字节1")
                  }
                }
                n6565 = Build Array(w16770, w16769) -> (w16768:i32[])
              }
              frame 2 {
                # "电压不均衡"
                n6566 = disable-structure shown="启用" {
                  disable-tunnel: [w16785 w16788] -> w16781
                  disable-tunnel: [w16784 w16788] -> w16780
                  disable-tunnel: w16778 -> [w16783 _]
                  frame Disabled {
                    n6567 = Unbundle By Name(w16783) -> ("电压不均衡(V)"=w16782:dbl)
                    n6568 = call "输入分辨率计算-EV05.vi"("1字节?"=FALSE, "数值"=w16782, "分辨率"=0.1) -> ("低字节"=w16784:dbl, "高字节1"=w16785:dbl)  [unwired: 2 in, 5 out]
                  }
                  frame Enabled {
                    w16788 = 255 ("高字节1")
                  }
                }
                n6569 = Build Array(w16781, w16780) -> (w16779:i32[])
              }
              frame 3 {
                # "温度过高"
                n6570 = disable-structure shown="启用" {
                  disable-tunnel: [w16795 255 ("高字节1")] -> w16791
                  disable-tunnel: w16789 -> [w16793 _]
                  frame Disabled {
                    n6571 = Unbundle By Name(w16793) -> ("温度过高"=w16792:dbl)
                    n6572 = call "输入分辨率计算-EV05.vi"("1字节?"=TRUE, "数值"=w16792, "偏移量"=-40.0, "分辨率"=1.0) -> ("高字节1"=w16795:dbl)  [unwired: 1 in, 6 out]
                  }
                  frame Enabled {
                  }
                }
                n6573 = Build Array(w16791) -> (w16790:i32[])
              }
              frame 4 {
                # "温度过低"
                n6574 = disable-structure shown="启用" {
                  disable-tunnel: [w16805 255 ("高字节1")] -> w16801
                  disable-tunnel: w16799 -> [w16803 _]
                  frame Disabled {
                    n6575 = Unbundle By Name(w16803) -> ("温度过低"=w16802:dbl)
                    n6576 = call "输入分辨率计算-EV05.vi"("1字节?"=TRUE, "数值"=w16802, "偏移量"=-40.0, "分辨率"=1.0) -> ("高字节1"=w16805:dbl)  [unwired: 1 in, 6 out]
                  }
                  frame Enabled {
                  }
                }
                n6577 = Build Array(w16801) -> (w16800:i32[])
              }
              frame 5 {
                # "温度不均衡"
                n6578 = disable-structure shown="启用" {
                  disable-tunnel: [w16814 255 ("高字节1")] -> w16811
                  disable-tunnel: w16809 -> [w16813 _]
                  frame Disabled {
                    n6579 = Unbundle By Name(w16813) -> ("温度不均衡"=w16812:dbl)
                    n6580 = call "输入分辨率计算-EV05.vi"("1字节?"=TRUE, "数值"=w16812, "分辨率"=1.0) -> ("高字节1"=w16814:dbl)  [unwired: 2 in, 6 out]
                  }
                  frame Enabled {
                  }
                }
                n6581 = Build Array(w16811) -> (w16810:i32[])
              }
              frame 6 {
                # "SOC过低"
                n6582 = disable-structure shown="启用" {
                  disable-tunnel: w16820 -> [w16837 _]
                  disable-tunnel: [w16823 w16840] -> w16819
                  disable-tunnel: [w16822 w16840] -> w16818
                  frame Disabled {
                    n6583 = Unbundle By Name(w16837) -> ("SOC过低"=w16836:dbl)
                    n6584 = call "输入分辨率计算-EV05.vi"("1字节?"=FALSE, "数值"=w16836, "分辨率"=0.1) -> ("低字节"=w16825:dbl, "高字节1"=w16826:dbl)  [unwired: 2 in, 5 out]
                    n6585 = call "二进制解析-8.6.vi"("索引"=4, "数值"=0) -> ("低位子数组"=w16829:i32[])  [unwired: 3 out]
                    n6586 = call "二进制解析-8.6.vi"("索引"=4, "数值"=w16826) -> ("低位子数组"=w16832:i32[])  [unwired: 3 out]
                    n6587 = call "二进制解析-8.6.vi"("索引"=4, "数值"=w16825) -> ("低位子数组"=w16830:i32[], "高位子数组"=w16831:i32[])  [unwired: 2 out]
                    n6588 = Insert Into Array(array=w16832, new element=w16831) -> (w16834:i32[])  [unwired: 1 in]
                    n6589 = Insert Into Array(array=w16830, new element=w16829) -> (w16828:i32[])  [unwired: 1 in]
                    n6590 = call "数值二进制转十进制-8.6.vi"("子数组"=w16828) -> ("十进制数值"=w16823:i32)  [unwired: 4 out]
                    n6591 = call "数值二进制转十进制-8.6.vi"("子数组"=w16834) -> ("十进制数值"=w16822:i32)  [unwired: 4 out]
                  }
                  frame Enabled {
                    w16840 = 255 ("高字节1")
                  }
                }
                n6592 = Build Array(w16818, w16819) -> (w16821:i32[])
              }
            }
            n6593 = Insert Into Array(array=w16752, new element=w16751) -> (w16753:dbl[])  [unwired: 1 in]
          }
          n6594 = Build Array(w16746) -> (w16745:dbl[][])
        }
        frame "电压过高(3)" {
          n6595 = Unbundle By Name(w16845) -> ("三级故障(从板)"=w16846:refnum<vi>)
          n6596 = property class="Clust (严格)"(reference=w16846) -> ("Value"=w16844:T8)  [unwired: 1 in, 2 out]
          n6597 = for {
            N: 7 -> [_]
            tunnel: w16844 -> [w16856]
            shift-right: [w16855] -> w16848
            shift-left: dbl[] [] -> [w16854]
            i -> [w16857]
            n6598 = case shown="0, 默认" w16857 {
              tunnel: w16856 -> [w16858 w16869 w16880 w16891 w16901 w16911 w16922]
              tunnel: [w16859 w16870 w16881 w16892 w16902 w16912 w16923] -> w16853
              frame 0, Default {
                # "电压过高"
                n6599 = disable-structure shown="启用" {
                  disable-tunnel: [w16865 w16868] -> w16861
                  disable-tunnel: [w16864 w16868] -> w16860
                  disable-tunnel: w16858 -> [w16863 _]
                  frame Enabled {
                    n6600 = Unbundle By Name(w16863) -> ("电压过高"=w16862:dbl)
